vi "PTSequencer.ProcConstructor.vi"(0 "i ref in":refnum<vi>, 3 "ms timeout (10000)":i32=10000, 5 "error in (no error)":errorcluster) -> (14 "i ref out":refnum<vi>, 17 "timed out":bool, 19 "error out":errorcluster)   [LabVIEW 2014, in "PTSequencer.lvlib"]
uses:
  PTSequencer.lvlib
  CSlibraries-extern/DimLVEvent/LVDimInterface/LVDimInterface.lvlib
  CSCore/CSSystem/CSSystemLib/CSSystemLib.lvlib
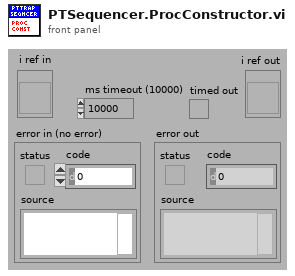
[diagram p1: front panel]
types:
  T1 = typedef "PTSequencer.lvlib/PTSequencer.i attribute.ctl" = cluster{"subsequence":bool, "mode":T2, "i step":i32, "nofLoops":i32, "i loop":i32, "Running":bool, "Paused":bool, "step done":bool, "loop done":bool, "seq done":bool, "DIM IDs":cluster{"step done":i32, "loop done":i32, "seq done":i32, "i step":i32, "i loop":i32}, "use stop conditions":bool, "stop conditions":T3[], "Step List":T5[], "DIM subsriptions":string[], "stop cond indexes":i32[], "step cond indexes":cluster{"step condition IDs":cluster{"step ID":i32, "condition ID":i32}[]}[], "Delay Start Time":timestamp, "status":string, "stopping":bool}
  T2 = typedef "PTSequencer.lvlib/PTSequencer.mode.ctl" = enum16{"single", "loop", "for loop"}
  T3 = typedef "PTSequencer.lvlib/PTSequencer.DIM service condition.ctl" = cluster{"DIM service":string, "descr":string, "nomValue":T4, "actValue":T4, "matched":bool, "DIM Status":cluster{"no link":bool, "quality":i32, "Time Stamp":timestamp}}
  T4 = typedef "CoreDefs.rawDataType.ctl" = i8[]
  T5 = typedef "PTSequencer.lvlib/PTSequencer.step.ctl" = cluster{"description":string, "object parameters":cluster{"object":string, "selector":string, "descriptor":string, "data":T4, "subsequence":bool, "call mode":enum16{"Simple DIM", "Synchronous"}, "data in":T4}, "result action":cluster{"check":bool, "passed":enum16{"Next", "Previous", "Repeat", "Jump"}, "failed":enum16{"Next", "Previous", "Repeat", "Jump"}, "jumpID_passed":i32, "jumpID_failed":i32}, "conditions":T3[], "fulfilled ":bool, "use delay":bool, "delay time (s)":dbl, "ID":i32}
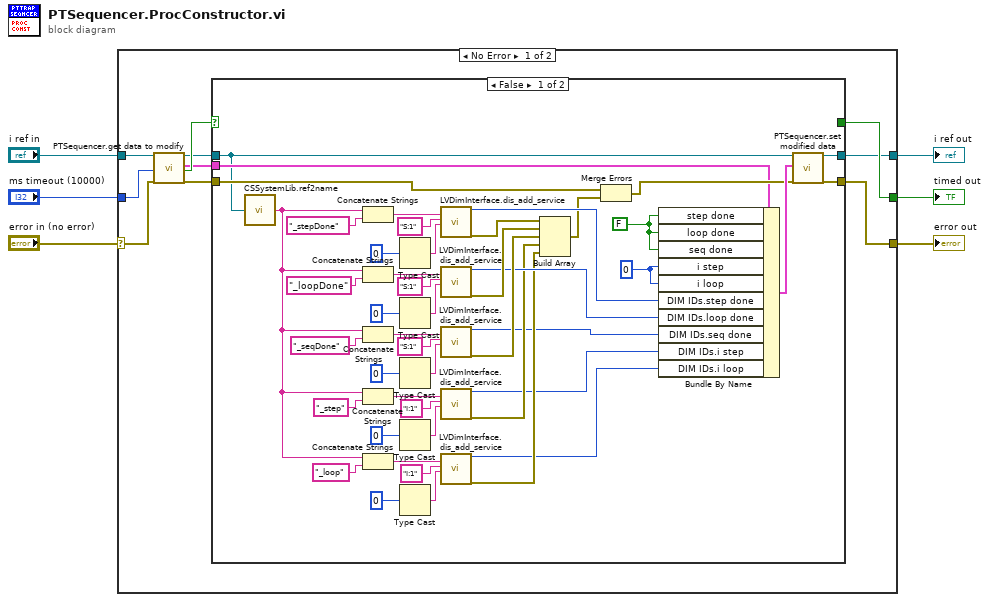
[diagram p0: block diagram]
diagram:
  n1 = case shown="No Error" "error in (no error)" {
    selector: "error in (no error)" -> [w12 w67]
    tunnel: [w9 w67] -> w5
    tunnel: "i ref in" -> [w16 w66]
    tunnel: "ms timeout (10000)" -> [w15 _]
    tunnel: [w13 _] -> w2
    tunnel: [w10 w66] -> w1
    frame No Error {
      n2 = call "PTSequencer.get data to modify.vi"("i ref in"=w16, "ms timeout (10000)"=w15, "error in (no error)"=w12) -> ("i ref out"=w11:refnum<vi>, "i attribute"=w7:T1, "timed out"=w14:bool, "error out"=w8:errorcluster)  [unwired: 13 in]
      n3 = case shown="False" w14 {
        selector: w14 -> [_ w65]
        tunnel: [_ w65] -> w13
        tunnel: w11 -> [w54 w63]
        tunnel: [w62 w63] -> w10
        tunnel: [w61 w64] -> w9
        tunnel: w8 -> [w57 w64]
        tunnel: w7 -> [w55 _]
        frame False {
          w50 = 0
          w52 = FALSE
          n4 = call "CSSystemLib.ref2name.vi"("obj refnum"=w54) -> ("name"=w23:string)
          n5 = Concatenate Strings(w23, "_stepDone" ("initial string")) -> (w59:string)
          n6 = Concatenate Strings(w23, "_loopDone" ("initial string")) -> (w48:string)
          n7 = Concatenate Strings(w23, "_seqDone" ("initial string")) -> (w43:string)
          n8 = Concatenate Strings(w23, "_step" ("initial string")) -> (w33:string)
          n9 = Concatenate Strings(w23, "_loop" ("initial string")) -> (w28:string)
          n10 = Type Cast(x=i16 0) -> (*(type *) &x=w51:string)  [unwired: 1 in]
          n11 = Type Cast(x=i16 0) -> (*(type *) &x=w45:string)  [unwired: 1 in]
          n12 = Type Cast(x=i16 0) -> (*(type *) &x=w40:string)  [unwired: 1 in]
          n13 = Type Cast(x=0) -> (*(type *) &x=w30:string)  [unwired: 1 in]
          n14 = Type Cast(x=0) -> (*(type *) &x=w25:string)  [unwired: 1 in]
          n15 = call "LVDimInterface.dis_add_service.vi"("serviceName"=w59, "typeDescriptor"="S:1" ("initial string"), "data"=w51) -> ("my_serviceID"=w35:i32, "error out"=w38:errorcluster)  [unwired: 15 in]
          n16 = call "LVDimInterface.dis_add_service.vi"("serviceName"=w48, "typeDescriptor"="S:1" ("initial string"), "data"=w45) -> ("my_serviceID"=w34:i32, "error out"=w37:errorcluster)  [unwired: 15 in]
          n17 = call "LVDimInterface.dis_add_service.vi"("serviceName"=w43, "typeDescriptor"="S:1" ("initial string"), "data"=w40) -> ("my_serviceID"=w20:i32, "error out"=w36:errorcluster)  [unwired: 15 in]
          n18 = call "LVDimInterface.dis_add_service.vi"("serviceName"=w33, "typeDescriptor"="I:1" ("initial string"), "data"=w30) -> ("my_serviceID"=w19:i32, "error out"=w22:errorcluster)  [unwired: 15 in]
          n19 = call "LVDimInterface.dis_add_service.vi"("serviceName"=w28, "typeDescriptor"="I:1" ("initial string"), "data"=w25) -> ("my_serviceID"=w18:i32, "error out"=w21:errorcluster)  [unwired: 15 in]
          n20 = Build Array(w38, w37, w36, w22, w21) -> (w17:errorcluster[])
          n21 = Merge Errors(w57, w17) -> (w56:errorcluster)
          n22 = Bundle By Name(cluster=w55, "step done"=w52, "loop done"=w52, "seq done"=w52, "i step"=w50, "i loop"=w50, "DIM IDs.step done"=w35, "DIM IDs.loop done"=w34, "DIM IDs.seq done"=w20, "DIM IDs.i step"=w19, "DIM IDs.i loop"=w18) -> (w60:T1)
          n23 = call "PTSequencer.set modified data.vi"("i ref in"=w54, "CLASS.i attribute"=w60, "error in (no error)"=w56) -> ("i ref out"=w62:refnum<vi>, "error out"=w61:errorcluster)  [unwired: 15 in]
        }
        frame True {
        }
      }
    }
    frame Error {
    }
  }
  "error out" <- w5
  "i ref out" <- w1
  "timed out" <- w2
